vi "SetVPB.vi"(1 "lines":u32, 2 "keep":u8, 3 "range":u32) -> ()   [LabVIEW 2014]
uses:
  ESLSCDLL.dll
panel:
  # "Set range for partial binning of FFT"
  # "range 1..5"
  # "lines per range"
  # "1 if range should be kept"
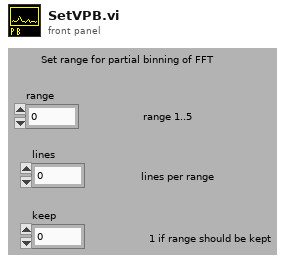
[diagram p1: front panel]
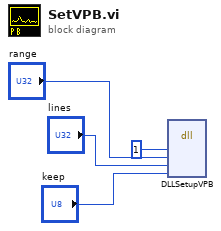
[diagram p0: block diagram]
diagram:
  n1 = dll-call lib="C:/Users/Gerhard/Documents/New64/lv/1cam/board.vis/ESLSCDLL.dll" fn="DLLSetupVPB" ("lwlscdll.dll:DLLRsTOREG")("drv"=u32 1, "range"="range", "lines"="lines", "keep"="keep") -> ()  [unwired: 8 in, 2 out]
